vi "Run Tests.vi"(8 "error in (no error)":errorcluster) -> (0 "error out":errorcluster)   [LabVIEW 2020]
uses:
  <vilib>/addons/_JKI Toolkits/Caraya/run-tests/Run Test (Scalar Path).vi
  <vilib>/addons/_JKI Toolkits/Caraya/Caraya.lvlib
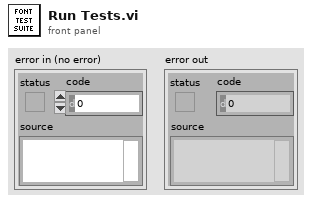
[diagram p1: front panel]
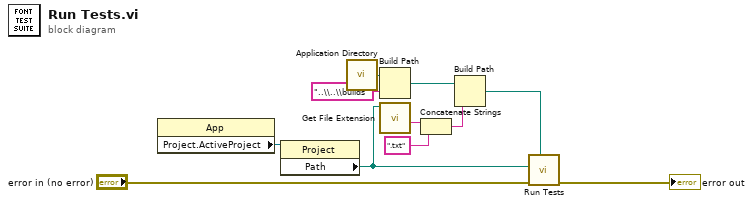
[diagram p0: block diagram]
diagram:
  n1 = property on="Property Node" class="App"() -> ("Project.ActiveProject"=w11:refnum<vi>)  [unwired: 2 in, 2 out]
  n2 = property on="Property Node" class="Project"(reference=w11) -> ("Path"=w10:path)  [unwired: 1 in, 2 out]
  n3 = call <vilib>:"Application Directory.vi"() -> ("Application Directory"=w3:path)
  n4 = Build Path(base path=w3, name or relative path="..\\..\\builds" ("string")) -> (appended path=w1:path)
  n5 = call <vilib>:"Get File Extension.vi"("file"=w10) -> ("filename without extension"=w9:string)  [unwired: 6 in, 4 out]
  n6 = Concatenate Strings(w9, ".txt" ("string")) -> (w8:string)
  n7 = Build Path(base path=w1, name or relative path=w8) -> (appended path=w6:path)
  n8 = call-poly <vilib>:"Run Tests.vi"("Report Path"=w6, "error in"="error in (no error)", "Test Path"=w10) -> ("error out"=→"error out":errorcluster)  [unwired: 8 in]
